vi "Decorator.vi"(10 "Actor":refnum<class "Actor.lvclass">, 11 "jettl Queue Actor in":refnum<class "jettl Queue Actor.lvclass">) -> (3 "jettl Queue Actor out":refnum<class "jettl Queue Actor.lvclass">)   [LabVIEW 2021, in "jettl Queue Actor.lvlib" / "jettl Queue Actor.lvclass"]
uses:
  jettl Queue Actor.lvclass
  Actor/Actor/Actor.lvclass
  jettl Queue Actor.lvclass/jettl Queue Actor.ctl
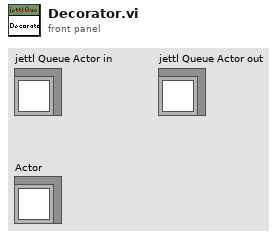
[diagram p1: front panel]
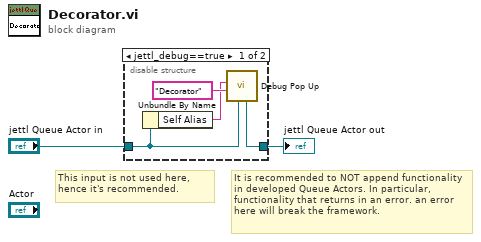
[diagram p0: block diagram]
diagram:
  # "It is recommended to NOT append functionality in developed Queue Actors. In particular, functionality that returns in an error. an error here will break the framework."
  # "This input is not used here, hence it's recommended."
  n1 = disable-structure shown="jettl_debug==true" {
    disable-tunnel: "jettl Queue Actor in" -> [w4 _]
    disable-tunnel: [w5 _] -> w1
    frame condition #0 (active) {
      n2 = Unbundle By Name(w4) -> ("Self Alias"=w3:string)
      n3 = call "Debug Pop Up.vi"("Input"=w4, "Method"="Decorator", "Alias"=w3) -> ("Output"=w5:refnum<class "jettl Queue Actor.lvclass">)  [unwired: 8 in]
    }
    frame condition #1 {
    }
  }
  "jettl Queue Actor out" <- w1
